vi "SubVI_RGBConvertTo1DArray.vi"(7 "i32PixelAmount":i32, 8 "au8Channel-R":u8[](array[numeric]), 9 "au8Channel-G":u8[](array[numeric]), 10 "au8Channel-B":u8[](array[numeric]), 11 "au8SerializedImage[in]":u8[](array[numeric])) -> (3 "au8SerializedImage[out]":u8[](array[numeric]))   [LabVIEW 2013]
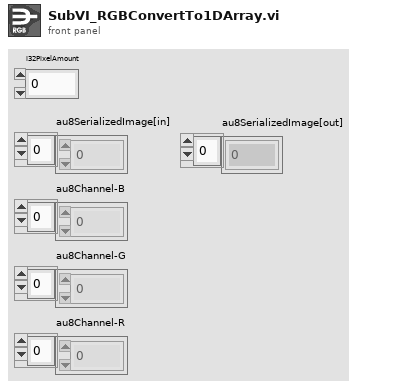
[diagram p1: front panel]
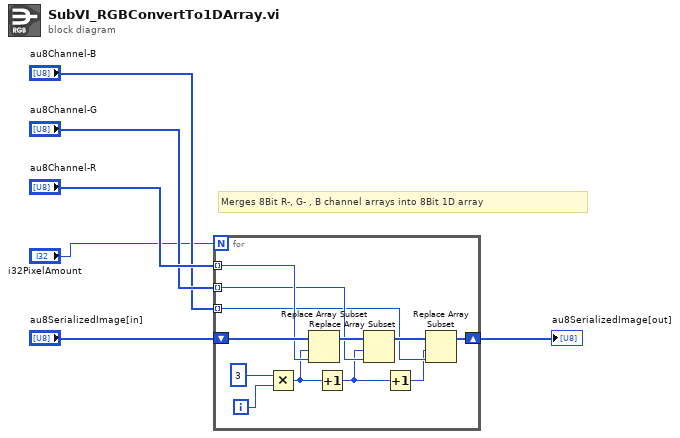
[diagram p0: block diagram]
diagram:
  # "Merges 8Bit R-, G- , B channel arrays into 8Bit 1D array"
  n1 = for "For-Schleife" {
    N: "i32PixelAmount" -> [_]
    tunnel: "au8Channel-R" -> [w14] mode=indexing
    tunnel: "au8Channel-G" -> [w13] mode=indexing
    tunnel: "au8Channel-B" -> [w12] mode=indexing
    shift-right: [w15] -> w2
    shift-left: "au8SerializedImage[in]" -> [w18]
    i -> [w11]
    n2 = Multiply(x=3, y=w11) -> (x*y=w9:i32)
    n3 = Replace Array Subset(array=w18, new element=w14, index=w9) -> (w17:u8[])
    n4 = Increment(x=w9) -> (x+1=w8:i32)
    n5 = Replace Array Subset(array=w17, new element=w13, index=w8) -> (w16:u8[])
    n6 = Increment(x=w8) -> (x+1=w7:i32)
    n7 = Replace Array Subset(array=w16, new element=w12, index=w7) -> (w15:u8[])
  }
  "au8SerializedImage[out]" <- w2
